vi "UpdateStatorResistance.vi"(11 "Motor Info In":T1) -> (3 "Motor Info Out":T1)   [LabVIEW 2017, in "McsaAnalysisFunctions.lvlib"]
uses:
  <vilib>/addons/InsightCM/Utilities/Analysis/MCSA/McsaAnalysisFunctions.lvlib
  <vilib>/addons/InsightCM/Utilities/Analysis/MCSA/controls/McsaMotor.ctl
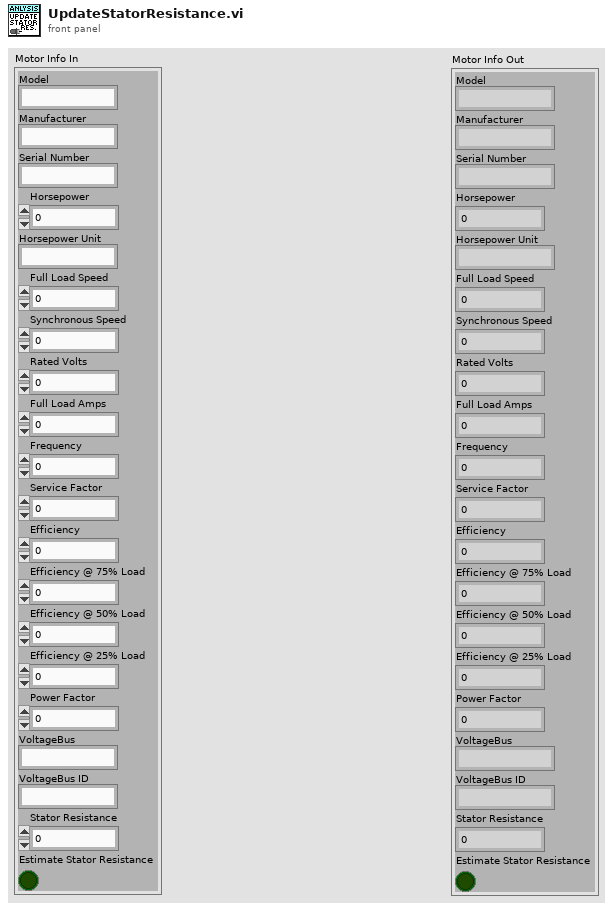
[diagram p1: front panel]
types:
  T1 = typedef "McsaAnalysisFunctions.lvlib/McsaMotor.ctl" = cluster{"Model":string, "Manufacturer":string, "Serial Number":string, "Horsepower":dbl, "Horsepower Unit":string, "Full Load Speed":dbl, "Synchronous Speed":dbl, "Rated Volts":dbl, "Full Load Amps":dbl, "Frequency":dbl, "Service Factor":dbl, "Efficiency":dbl, "Efficiency @ 75% Load":dbl, "Efficiency @ 50% Load":dbl, "Efficiency @ 25% Load":dbl, "Power Factor":dbl, "VoltageBus":string, "VoltageBus ID":string, "Stator Resistance":dbl, "Estimate Stator Resistance":bool}
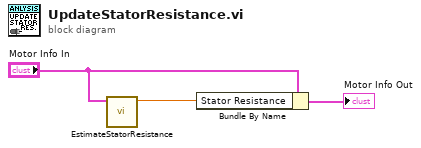
[diagram p0: block diagram]
diagram:
  n1 = call <vilib>:"EstimateStatorResistance.vi"("motor nameplate information"="Motor Info In") -> ("stator resisitance [ohms]"=w2:dbl)  [unwired: 10 in]
  n2 = Bundle By Name(cluster="Motor Info In", "Stator Resistance"=w2) -> (→"Motor Info Out":T1)
